vi "days since 1900.vi"(1 "seconds since 1904":dbl format="%.2f") -> (0 "Days":dbl format="%.2f")   [LabVIEW 2012]
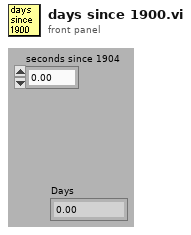
[diagram p1: front panel]
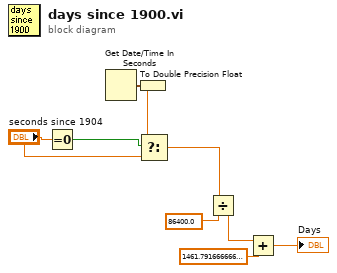
[diagram p0: block diagram]
diagram:
  n1 = Equal To 0?(x="seconds since 1904") -> (x = 0?=w3:bool)
  n2 = Get Date/Time In Seconds() -> (seconds since 1Jan1904=w1:timestamp)
  n3 = To Double Precision Float(number=w1) -> (double precision float=w5:dbl)
  n4 = Select(t=w5, s=w3, f="seconds since 1904") -> (s? t:f=w4:dbl)
  n5 = Divide(x=w4, y=86400.0) -> (x/y=w8:dbl)
  n6 = Add(x=w8, y=1461.7916666666667) -> (x+y=→"Days":dbl)
